vi "Unflatten Value.vi"(8 "Error In":errorcluster, 10 "Value":string, 11 "Bool Array In":refnum<class "1D Bool.lvclass">) -> (0 "Error Out":errorcluster, 3 "Bool Array Out":refnum<class "1D Bool.lvclass">)   [LabVIEW 2017, in "Tree API.lvlib" / "1D Bool.lvclass"]
uses:
  1D Bool.lvclass
  Tree Manager/Tree.lvclass
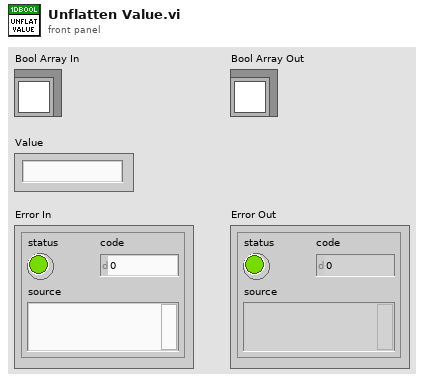
[diagram p1: front panel]
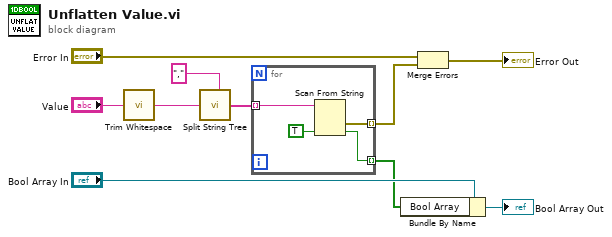
[diagram p0: block diagram]
diagram:
  n1 = call <vilib>:"Trim Whitespace.vi"("string"="Value") -> ("trimmed string"=w1:string)  [unwired: 1 in]
  n2 = call "Split String Tree.vi"("Split Pattern"="," ("Separator (,)"), "Input String"=w1) -> ("Split String"=w7:string[])  [unwired: 5 in]
  n3 = for {
    tunnel: w7 -> [w14] mode=indexing
    tunnel: [w12] -> w6 mode=indexing
    tunnel: [w11] -> w5 mode=indexing
    n4 = Scan From String(input string=w14, default 1=TRUE) -> (error out=w11:errorcluster, output 1=w12:bool)  [unwired: 3 in, 2 out]
  }
  n5 = Bundle By Name(cluster="Bool Array In", "Bool Array"=w6) -> (→"Bool Array Out":refnum<class "1D Bool.lvclass">)
  n6 = Merge Errors("Error In", w5) -> (→"Error Out":errorcluster)
